vi "Modify Standard Waveform.vi"(11 "Standard Wfm Config":T1={"Waveform Type"=0, "Sample Rate (Hz)"=10000000.0, "Frequency (Hz)"=10000.0, "Amplitude"=1.0, "Number of Cycles"=1, "Ramp Start"=0.0, "Ramp Stop"=1.0, "Length (s)"=0.001, "DC Value"=0.0, "Duration (s)"=0.001, "Pre Delay (s)"=0.0, "Post Delay (s)"=0.0}) -> (2 "Waveform Modified?":bool, 3 "Modified Waveform":waveform(dbl))   [LabVIEW 2025, in "TDMS Waveform Creator UI.lvlib"]
uses:
  TDMS Waveform Creator UI.lvlib
panel:
  in  "Post Delay (s)":dbl min=0.0 format="%#_6p"
  in  "Pre Delay (s)":dbl min=0.0 format="%#_6p"
  out "Waveform Name":string
  in  "Cancel":bool
  in  "OK":bool
  out "Actual Sample Size":i32
  out "Actual Duration (s)":dbl format="%#_6p"
  out "Waveform Preview":waveform(dbl)(graph)
  in  "Sample Rate (Hz)":dbl=10000000.0 min=0.0 format="%#_6p"
  in  "Config Type":enum32{"Periodic", "Ramp", "DC"}(tab)
  in  "Number of Cycles":u32=1 min=1
  in  "Frequency (Hz)":dbl=10000.0 format="%#_6p"
  in  "Amplitude":dbl=1.0
  in  "Ramp Start":dbl
  in  "Ramp Stop":dbl=1.0
  in  "Length (s)":dbl=0.001 format="%#_6p"
  in  "DC Value":dbl format="%#_6p"
  in  "Duration (s)":dbl=0.001 format="%#_6p"
  in  "Waveform Type":i32(listbox)
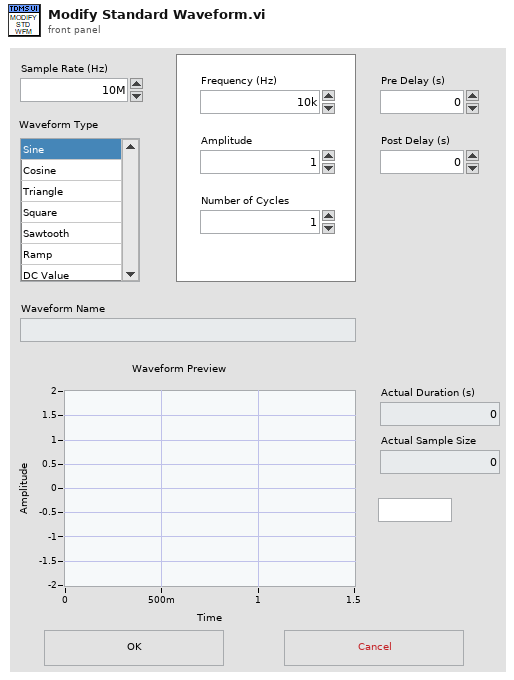
[diagram p1: front panel]
types:
  T1 = cluster{"Waveform Type":i32, "Sample Rate (Hz)":dbl, "Frequency (Hz)":dbl, "Amplitude":dbl, "Number of Cycles":u32, "Ramp Start":dbl, "Ramp Stop":dbl, "Length (s)":dbl, "DC Value":dbl, "Duration (s)":dbl, "Pre Delay (s)":dbl, "Post Delay (s)":dbl}
  T2 = enum16{"Ready", "Update Wfm", "Suggest Name Update"}
  T3 = enum8{"Enabled", "Disabled", "Disabled and Grayed Out"}
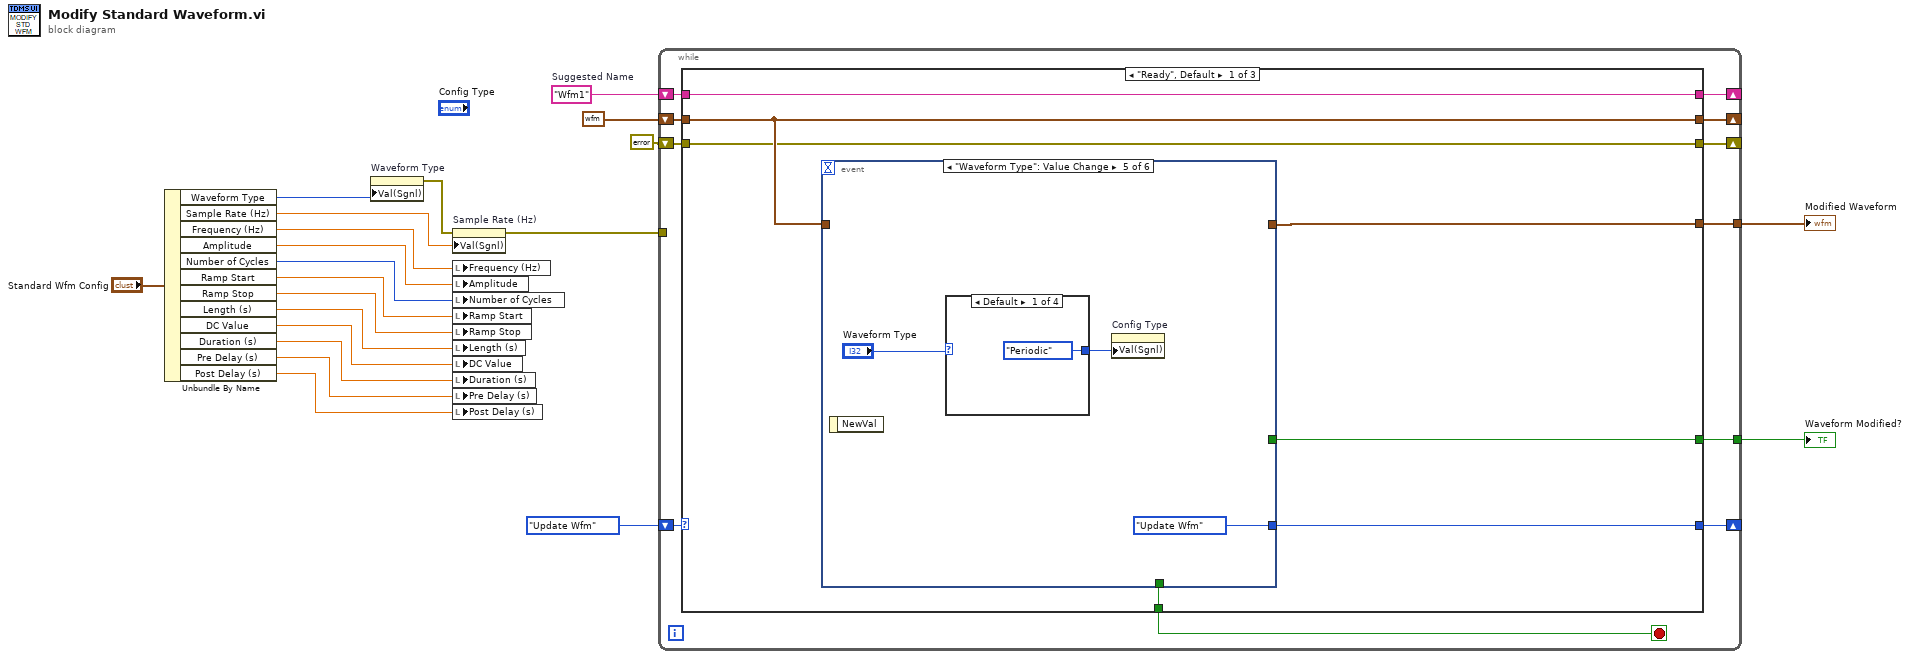
[diagram p0: block diagram]
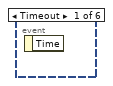
[diagram p2: hidden frame]
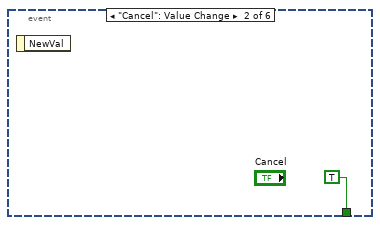
[diagram p3: hidden frame]
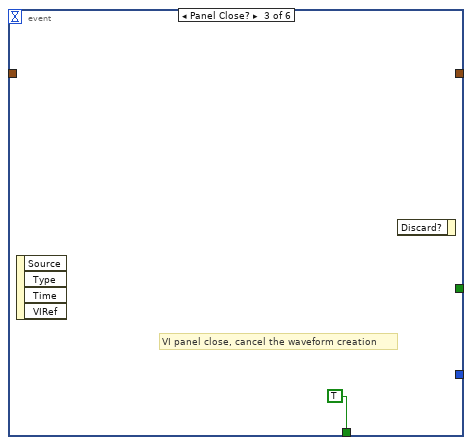
[diagram p4: hidden frame]
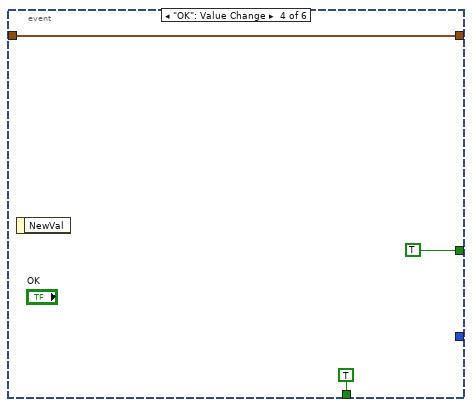
[diagram p5: hidden frame]
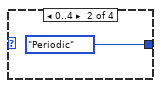
[diagram p6: hidden frame]
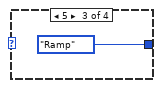
[diagram p7: hidden frame]
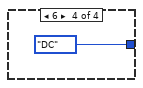
[diagram p8: hidden frame]
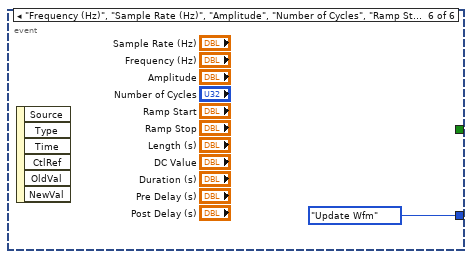
[diagram p9: hidden frame]
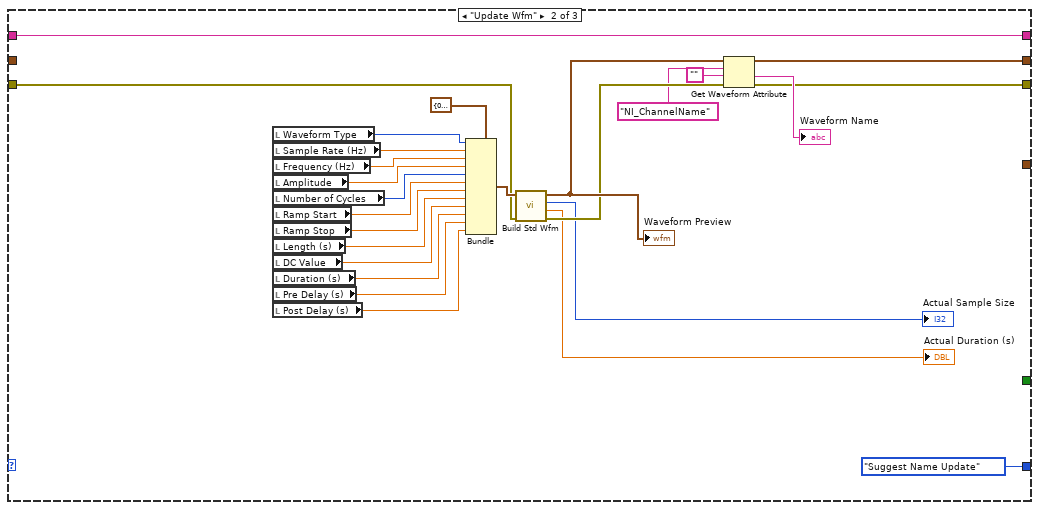
[diagram p10: hidden frame]
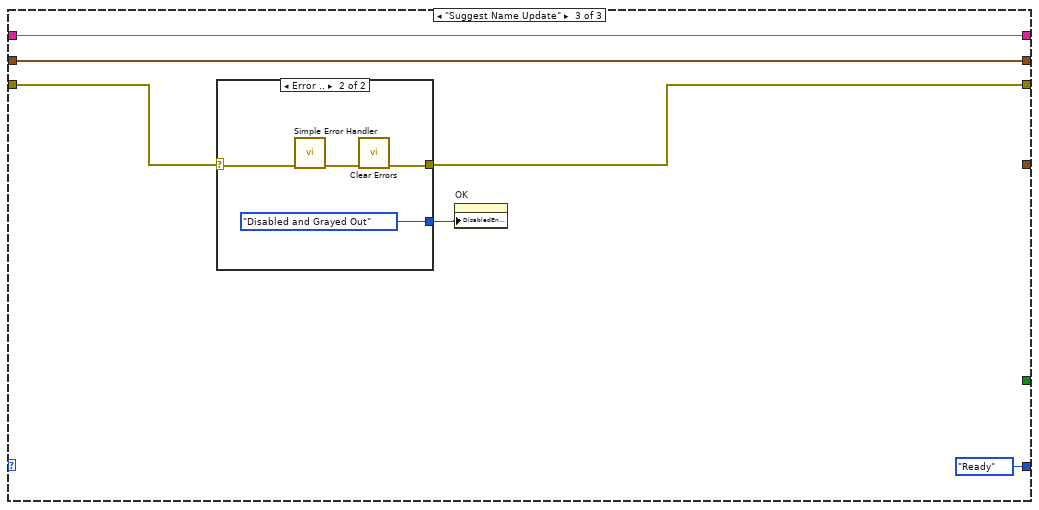
[diagram p11: hidden frame]
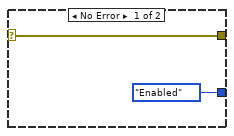
[diagram p12: hidden frame]
diagram:
  w19 = "Wfm1"  # Suggested Name
  n1 = Unbundle By Name("Standard Wfm Config") -> ("Waveform Type"=w13:i32, "Sample Rate (Hz)"=w12:dbl, "Frequency (Hz)"=w10:dbl, "Amplitude"=w9:dbl, "Number of Cycles"=w8:u32, "Ramp Start"=w7:dbl, "Ramp Stop"=w6:dbl, "Length (s)"=w5:dbl, "DC Value"=w4:dbl, "Duration (s)"=w3:dbl, "Pre Delay (s)"=w2:dbl, "Post Delay (s)"=w1:dbl)
  n2 = property on="Waveform Type" class="LstBox (strict)"("Val(Sgnl)"=w13) -> (error out=w11:errorcluster)  [unwired: 2 in, 1 out]
  n3 = property on="Sample Rate (Hz)" class="DigNum (strict)"(error in=w11, "Val(Sgnl)"=w12) -> (error out=w16:errorcluster)  [unwired: 1 in, 1 out]
  n4 = local write "Frequency (Hz)"(w10) -> ()
  n5 = local write "Amplitude"(w9) -> ()
  n6 = local write "Number of Cycles"(w8) -> ()
  n7 = local write "Ramp Start"(w7) -> ()
  n8 = local write "Ramp Stop"(w6) -> ()
  n9 = local write "Length (s)"(w5) -> ()
  n10 = local write "DC Value"(w4) -> ()
  n11 = local write "Duration (s)"(w3) -> ()
  n12 = local write "Pre Delay (s)"(w2) -> ()
  n13 = local write "Post Delay (s)"(w1) -> ()
  n14 = while {
    tunnel: [w31] -> w21
    shift-right: [w29] -> _
    shift-left: T2."Update Wfm" -> [w30]
    shift-right: [w27] -> _
    shift-left: w19 -> [w28]
    shift-right: [w25] -> _
    shift-left: waveform(dbl) {"t0"=timestamp(0 s since 1904-01-01), "dt"=1.0, "Y"=[]} ("Output Waveform") -> [w26]
    tunnel: [w24] -> w17
    tunnel: w16 -> [_]
    shift-right: [w23] -> _
    shift-left: errorcluster {"status"=FALSE, "code"=0, "source"=""} ("error out") -> [w22]
    stop <- w32 stop-if-true
    n15 = case shown="\"Ready\", Default" w30 {
      tunnel: [w39 _ _] -> w32
      tunnel: [w38 _ _] -> w31
      tunnel: [w37 T2."Suggest Name Update" T2."Ready"] -> w29
      tunnel: w28 -> [w36 w63 w82]
      tunnel: [w36 w63 w82] -> w27
      tunnel: w26 -> [w35 _ w84]
      tunnel: [w35 w62 w84] -> w25
      tunnel: [w34 _ _] -> w24
      tunnel: [w33 w57 w80] -> w23
      tunnel: w22 -> [w33 w56 w81]
      frame "Ready", Default {
        n16 = event shown="[4] \"Waveform Type\": Value Change" {
          selector: _ -> [_ _ _ _ _ _]
          dyn-events: _ -> [_ _ _ _ _ _]
          timeout: _ -> [_ _ _ _ _ _]
          tunnel: [_ TRUE TRUE TRUE _ _] -> w39
          tunnel: [_ _ _ TRUE _ _] -> w38
          tunnel: [_ _ _ _ T2."Update Wfm" T2."Update Wfm"] -> w37
          tunnel: w35 -> [_ _ _ w42 _ _]
          tunnel: [_ _ _ w42 _ _] -> w34
          event Timeout {
            n17 = event-data() -> ()  [unwired: 1 in, 1 out]
          }
          event "Cancel": Value Change {
            n18 = event-data() -> ()  [unwired: 1 in, 1 out]
          }
          event Panel Close? {
            # "VI panel close, cancel the waveform creation"
            n19 = event-data() -> ()  [unwired: 1 in, 4 out]
            n20 = event-data() -> ()  [unwired: 2 in, 1 out]
          }
          event "OK": Value Change {
            n21 = event-data() -> ()  [unwired: 1 in, 1 out]
          }
          event "Waveform Type": Value Change {
            n22 = event-data() -> ()  [unwired: 1 in, 1 out]
            n23 = case shown="Default" "Waveform Type" {
              tunnel: [enum32{"Periodic", "Ramp", "DC"}."Periodic" ("Value (Signaling)") enum32{"Periodic", "Ramp", "DC"}."Periodic" ("Value (Signaling)") enum32{"Periodic", "Ramp", "DC"}."Ramp" ("Value (Signaling)") enum32{"Periodic", "Ramp", "DC"}."DC" ("Value (Signaling)")] -> w47
              frame Default {
              }
              frame 0..4 {
              }
              frame 5 {
              }
              frame 6 {
              }
            }
            n24 = property on="Config Type" class="TabCtl (strict)"("Val(Sgnl)"=w47) -> ()  [unwired: 2 in, 2 out]
          }
          event "Frequency (Hz)", "Sample Rate (Hz)", "Amplitude", "Number of Cycles", "Ramp Start", "Ramp Stop", "Length (s)", "Duration (s)", "DC Value", "Pre Delay (s)", "Post Delay (s)": Value Change {
            n25 = event-data() -> ()  [unwired: 1 in, 6 out]
          }
        }
      }
      frame "Update Wfm" {
        n26 = local read "Waveform Type"() -> (w53:i32)
        n27 = local read "Sample Rate (Hz)"() -> (w77:dbl)
        n28 = local read "Frequency (Hz)"() -> (w76:dbl)
        n29 = local read "Amplitude"() -> (w75:dbl)
        n30 = local read "Number of Cycles"() -> (w74:u32)
        n31 = local read "Ramp Start"() -> (w73:dbl)
        n32 = local read "Ramp Stop"() -> (w72:dbl)
        n33 = local read "Length (s)"() -> (w71:dbl)
        n34 = local read "DC Value"() -> (w70:dbl)
        n35 = local read "Duration (s)"() -> (w69:dbl)
        n36 = local read "Pre Delay (s)"() -> (w68:dbl)
        n37 = local read "Post Delay (s)"() -> (w67:dbl)
        n38 = Bundle(cluster=T1 {"Waveform Type"=0, "Sample Rate (Hz)"=10000000.0, "Frequency (Hz)"=2000.0, "Amplitude"=1.0, "Number of Cycles"=1, "Ramp Start"=0.0, "Ramp Stop"=1.0, "Length (s)"=0.001, "DC Value"=0.0, "Duration (s)"=0.001, "Pre Delay (s)"=0.0, "Post Delay (s)"=0.0} ("Standard Wfm Config"), "Waveform Type"=w53, "Sample Rate (Hz)"=w77, "Frequency (Hz)"=w76, "Amplitude"=w75, "Number of Cycles"=w74, "Ramp Start"=w73, "Ramp Stop"=w72, "Length (s)"=w71, "DC Value"=w70, "Duration (s)"=w69, "Pre Delay (s)"=w68, "Post Delay (s)"=w67) -> (w66:T1)
        n39 = call "Build Std Wfm.vi"("error in"=w56, "Standard Wfm Config"=w66) -> ("error out"=w61:errorcluster, "Actual Duration (s)"=→"Actual Duration (s)":dbl, "Actual Sample Size"=→"Actual Sample Size":i32, "Waveform"=w64:waveform(dbl))  [unwired: 6 in]
        "Waveform Preview" <- w64
        n40 = Get Waveform Attribute(4:w61, 5:"", 6:"NI_ChannelName" ("name"), 7:w64) -> (0:w57:errorcluster, 1:→"Waveform Name":string, 3:w62:waveform(dbl))  [unwired: 1 out]
      }
      frame "Suggest Name Update" {
        n41 = case shown="Error .." w81 {
          selector: w81 -> [w86 w90]
          tunnel: [w86 w87] -> w80
          tunnel: [T3."Enabled" ("DisabledEnum") T3."Disabled and Grayed Out" ("DisabledEnum")] -> w79
          frame No Error {
          }
          frame Error {
            n42 = call <vilib>:"Simple Error Handler.vi"("error in (no error)"=w90) -> ("error out"=w89:errorcluster)  [unwired: 4 in, 4 out]
            n43 = call <vilib>:"Clear Errors.vi"("error in (no error)"=w89) -> ("error out"=w87:errorcluster)  [unwired: 5 in, 1 out]
          }
        }
        n44 = property on="OK" class="Bool"("DisabledEnum"=w79) -> ()  [unwired: 2 in, 2 out]
      }
    }
  }
  "Waveform Modified?" <- w21
  "Modified Waveform" <- w17
